vi "Dynamic Block Lock 2k.vi"(9 "Dynamic Block Lock Page Section 1K":T1, 11 "PN532 COM Port":refnum<visa-resource-name>) -> (0 "Error out":errorcluster, 2 "Succeeded":bool, 3 "PN532 COM Port Out":refnum<visa-resource-name>)   [LabVIEW 2012, in "NFC Driver.lvlib"]
uses:
  NFC Driver.lvlib
  Typedef/Dynamic Block Lock Page Section 1K.ctl
panel:
  out "result string":string
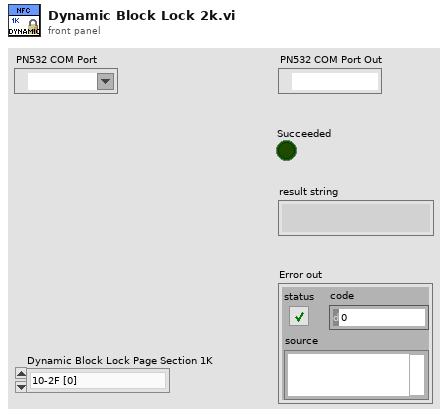
[diagram p1: front panel]
types:
  T1 = typedef "NFC Driver.lvlib/Dynamic Block Lock Page Section 1K.ctl" = enum16{"10-2F [0]", "30-4F [1]", "50-6F [2]", "70-8F [3]", "90-AF [4]", "B0-CF [5]", "D0-E1 [6]"}
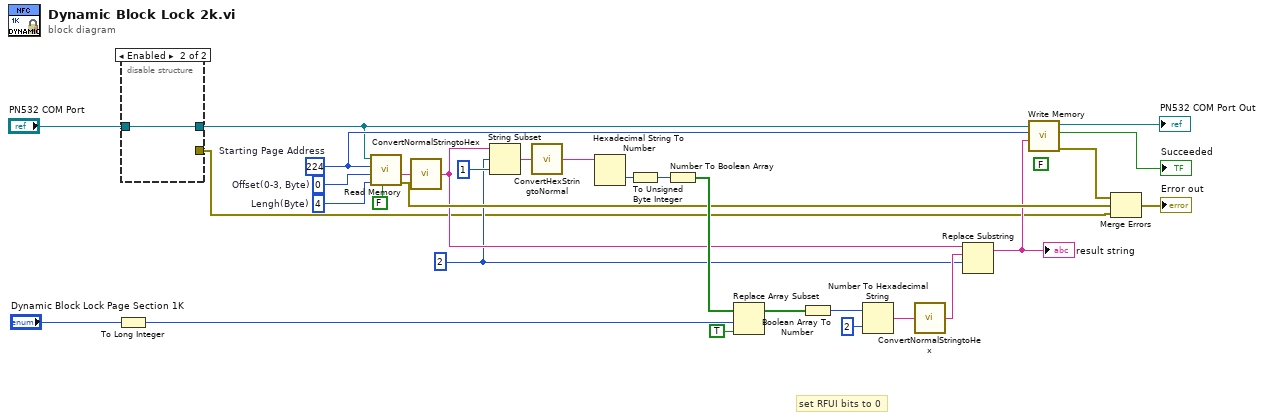
[diagram p0: block diagram]
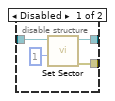
[diagram p2: hidden frame]
diagram:
  w7 = 2 ("offset (0)")
  w8 = 0  # Offset(0-3, Byte)
  (unwired) FALSE ("Data in ASCII")
  w28 = 4  # Lengh(Byte)
  w14 = 224  # Starting Page Address
  # "set RFUI bits to 0"
  n1 = To Long Integer(number="Dynamic Block Lock Page Section 1K") -> (32bit integer=w11:i32)
  n2 = disable-structure shown="Enabled" {
    disable-tunnel: "PN532 COM Port" -> [w34 w35]
    disable-tunnel: [w33 w35] -> w5
    disable-tunnel: [w31 _] -> w4
    frame Disabled {
      n3 = call "Set Sector.vi"("Numeric"=1, "PN532 COM Port"=w34) -> ("Error Out"=w31:errorcluster, "PN532 COM out"=w33:refnum<visa-resource-name>)  [unwired: 8 in]
    }
    frame Enabled {
    }
  }
  n4 = call "Read Memory.vi"("Reverse Output[F]"=FALSE, "length (Byte, max. 16)"=w28, "offset (Byte, max. 16)"=w8, "Page Address"=w14, "PN532 COM Port"=w5) -> ("error out"=w22:errorcluster, "Selected substring (HEX)"=w3:string)  [unwired: 2 in, 3 out]
  n5 = call "ConvertNormalStringtoHex.vi"("Normal String"=w3) -> ("Hex String"=w13:string)
  n6 = String Subset(string=w13, offset (0)=w7, length (rest)=1 ("length (rest)")) -> (substring=w16:string)
  n7 = call "ConvertHexStringtoNormal.vi"("Hex String"=w16) -> ("Normal String"=w15:string)
  n8 = Hexadecimal String To Number(string=w15) -> (number=w27:u32)  [unwired: 2 in, 1 out]
  n9 = To Unsigned Byte Integer(number=w27) -> (unsigned 8bit integer=w18:u8)
  n10 = Number To Boolean Array(number=w18) -> (Boolean array=w26:bool[])
  n11 = Replace Array Subset(array=w26, new element=TRUE ("new element/subarray"), index=w11) -> (w21:bool[])
  n12 = Boolean Array To Number(Boolean array=w21) -> (number=w25:u32)
  n13 = Number To Hexadecimal String(1:i16 2 ("width (-)"), 2:w25) -> (0:w12:string)
  n14 = call "ConvertNormalStringtoHex.vi"("Normal String"=w12) -> ("Hex String"=w9:string)
  n15 = Replace Substring(3:w7, 4:w9, 5:w13) -> (1:w10:string)  [unwired: 1 in, 1 out]
  "result string" <- w10
  n16 = call "Write Memory.vi"("Data to write (HEX, max 16 bytes)"=w10, "Page Address"=w14, "PN532 COM Port"=w5) -> ("Error Out"=w23:errorcluster, "Succesful?"=→"Succeeded":bool, "PN532 COM Port Out"=→"PN532 COM Port Out":refnum<visa-resource-name>)  [unwired: 6 in]
  n17 = Merge Errors(w23, w22, w4) -> (→"Error out":errorcluster)
